vi "Read Interactive.vi"(8 "error in (no error)":errorcluster, 11 "DefineSuite in":refnum<class "DefineSuite.lvclass">) -> (0 "error out":errorcluster, 2 "Interactive":bool, 3 "DefineSuite out":refnum<class "DefineSuite.lvclass">)   [LabVIEW 2021, in "Bananas.lvlib" / "DefineSuite.lvclass"]
uses:
  DefineSuite.lvclass
  DefineSuite.lvclass/DefineSuite.ctl
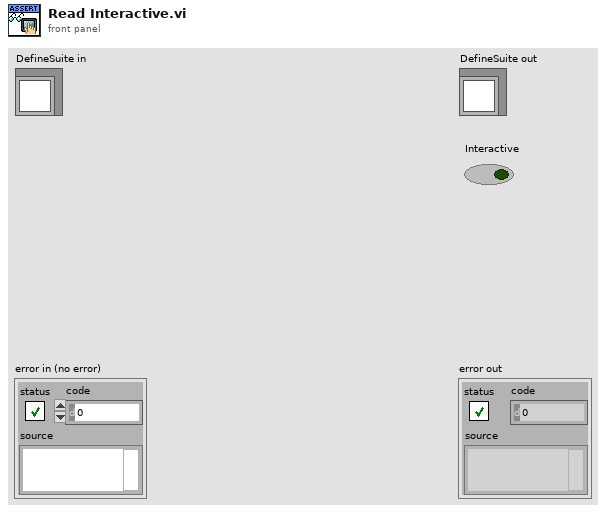
[diagram p1: front panel]
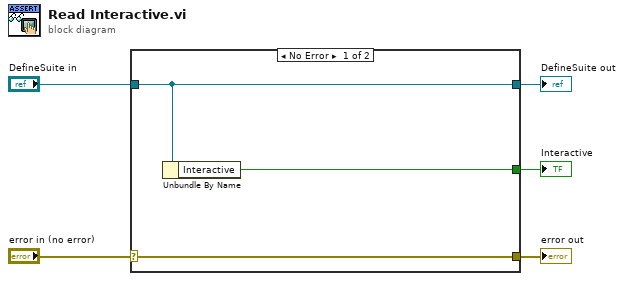
[diagram p0: block diagram]
diagram:
  n1 = case shown="No Error" "error in (no error)" {
    selector: "error in (no error)" -> [w8 w9]
    tunnel: [w8 w9] -> w4
    tunnel: [w7 w10] -> w2
    tunnel: "DefineSuite in" -> [w7 w10]
    tunnel: [w6 _] -> w1
    frame No Error {
      n2 = Unbundle By Name(w7) -> ("Interactive"=w6:bool)
    }
    frame Error {
    }
  }
  "error out" <- w4
  "DefineSuite out" <- w2
  "Interactive" <- w1
